vi "Linecut Example.vi"() -> ()   [LabVIEW 2016, in "graph_utilities.lvclass"]
uses:
  graph_utilities.lvclass
  graph_utilities.lvclass/graph_utilities.ctl
panel:
  in  "OK":bool
  in  "width (horizontal) 2":dbl=0.2
  in  "width (vertical) 2":dbl=0.2
  out "Horizontal 2":cluster{"Array":dbl[], "A x Vector":dbl[]}[](graph)
  out "Vertical 2":cluster{"Array":dbl[], "A x Vector":dbl[]}[](graph)
  in  "V2f 2":dbl[][](graph)=array73x213[15549 elements]
  in  "width (horizontal)":dbl=0.2
  in  "width (vertical)":dbl=0.2
  out "Horizontal":cluster{"Intensity Data":dbl[], "Array":dbl[]}[](graph)
  out "Vertical":cluster{"Array":dbl[], "A x Vector":dbl[]}[](graph)
  in  "V2f":dbl[][](graph)=array73x221[16133 elements]
  # "Control Graph:"
  # "Target:"
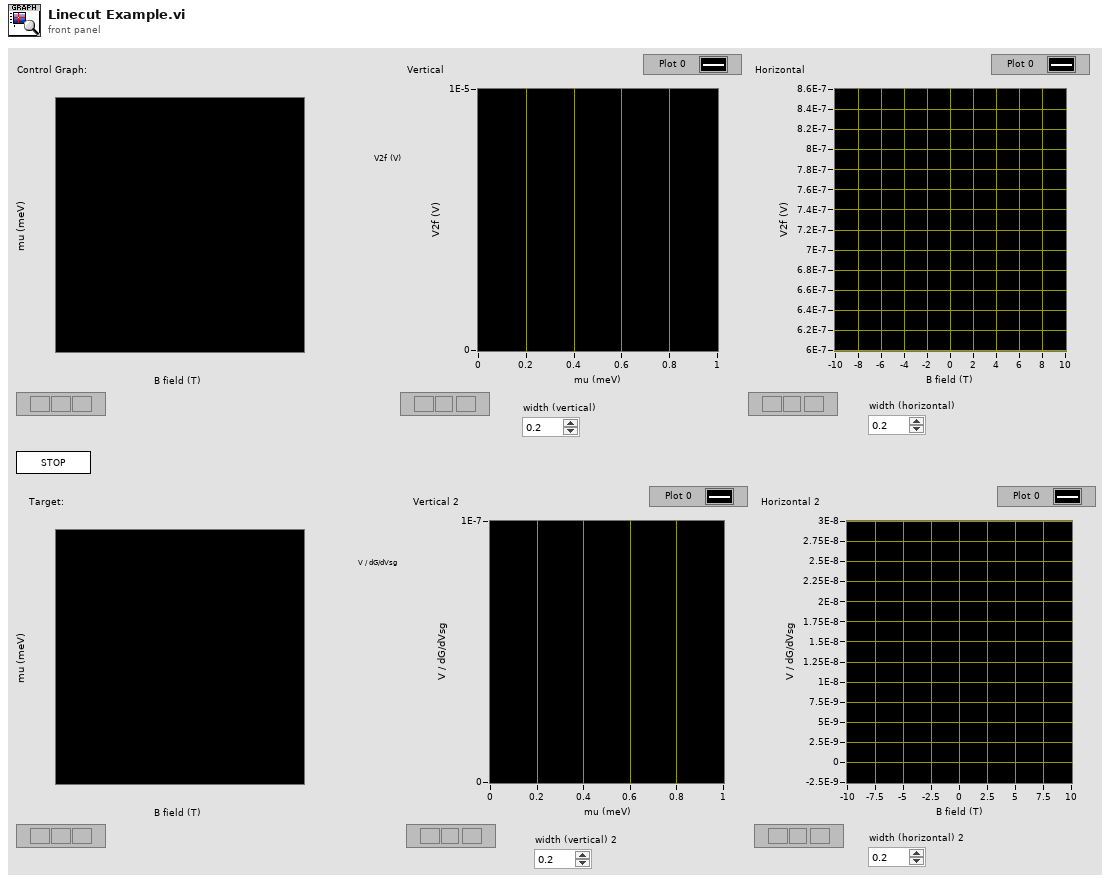
[diagram p1: front panel]
types:
  T1 = enum32{"Invalid", "Standard", "Closed", "Hidden", "Minimized", "Maximized"}
  T2 = enum32{"invalid app kind", "Development System", "Run Time System", "Student Edition", "Embedded LabVIEW", "Evaluation", "Custom"}
  T3 = cluster{"Core":cluster{"Current VI Reference":refnum<vi>, "Close Panel on Exit?":bool}, "graphs":refnum<class "graph_utilities.lvclass">[]}
  T4 = cluster{"Current VI Reference":refnum<vi>, "Close Panel on Exit?":bool}
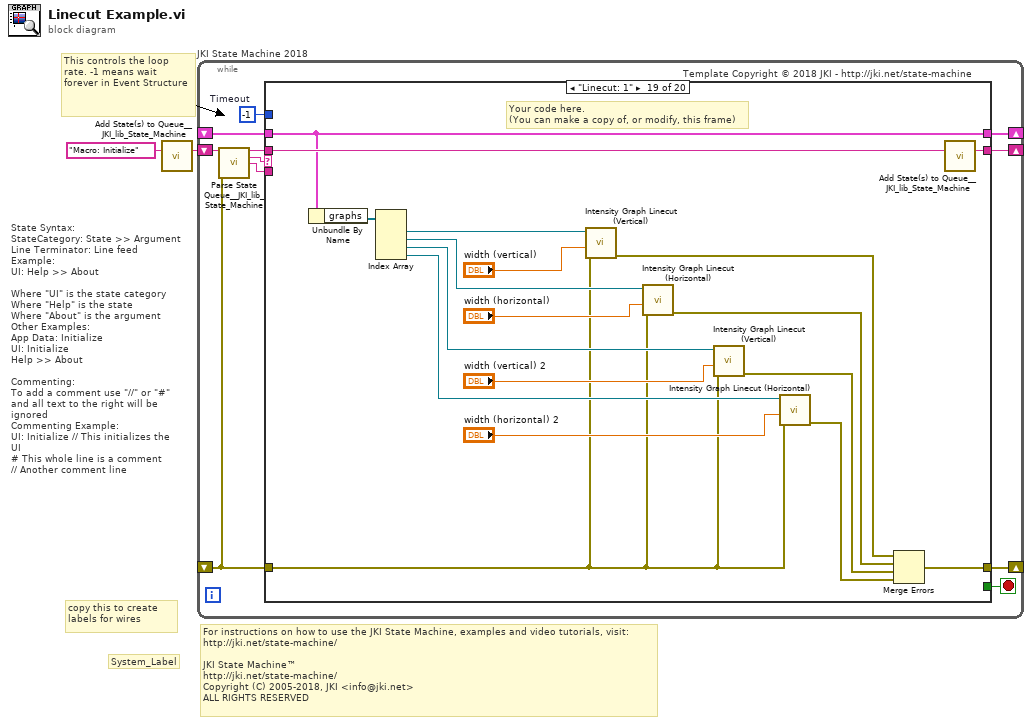
[diagram p0: block diagram]
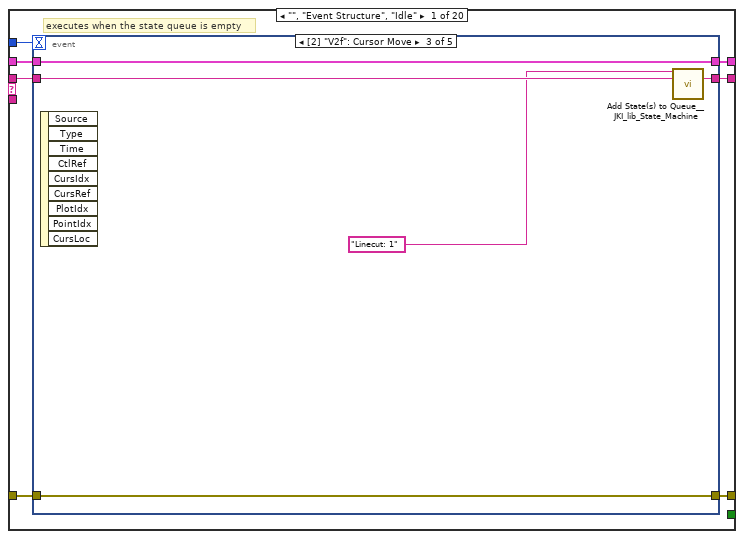
[diagram p2: hidden frame]
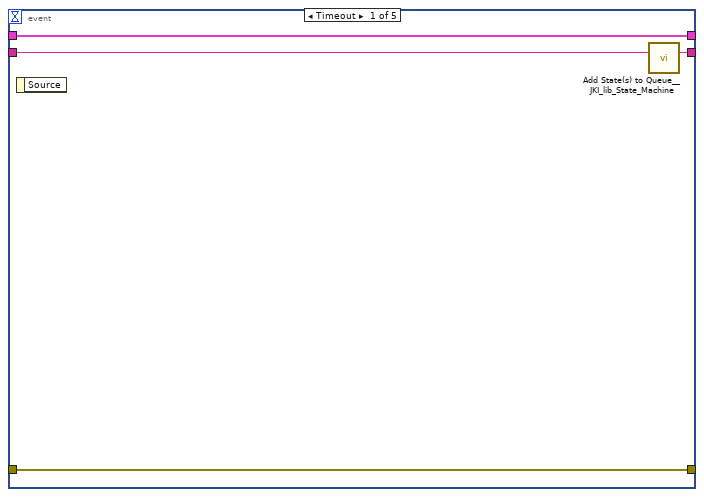
[diagram p3: hidden frame]
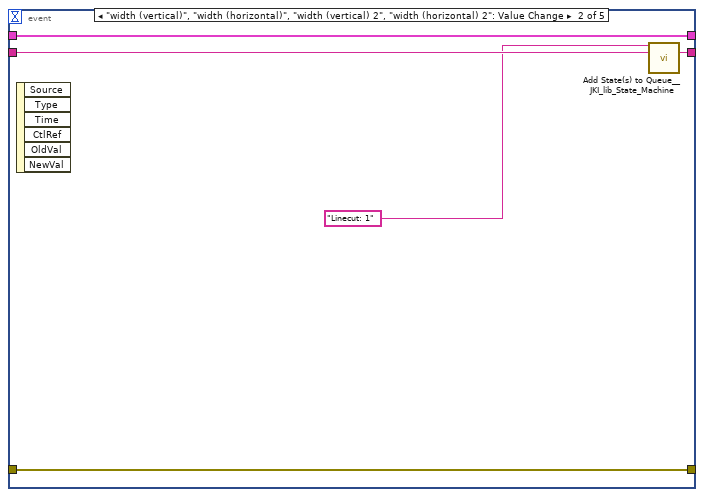
[diagram p4: hidden frame]
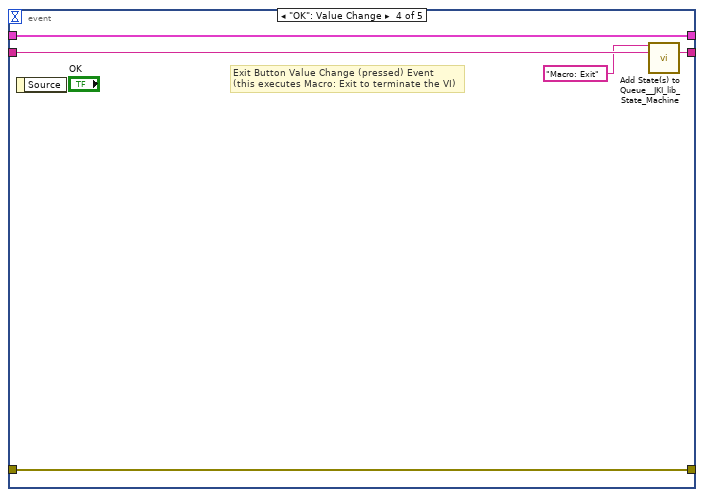
[diagram p5: hidden frame]
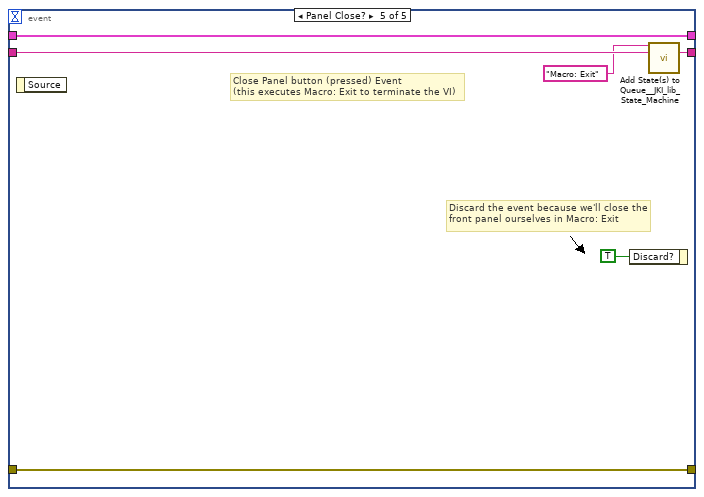
[diagram p6: hidden frame]
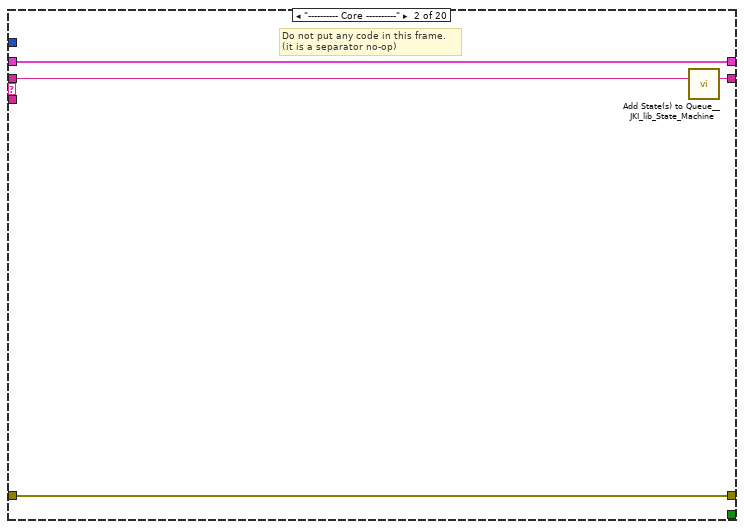
[diagram p7: hidden frame]
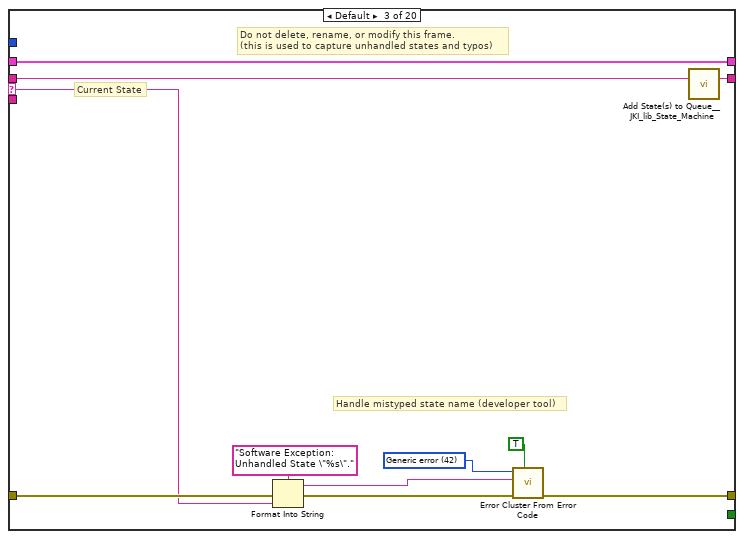
[diagram p8: hidden frame]
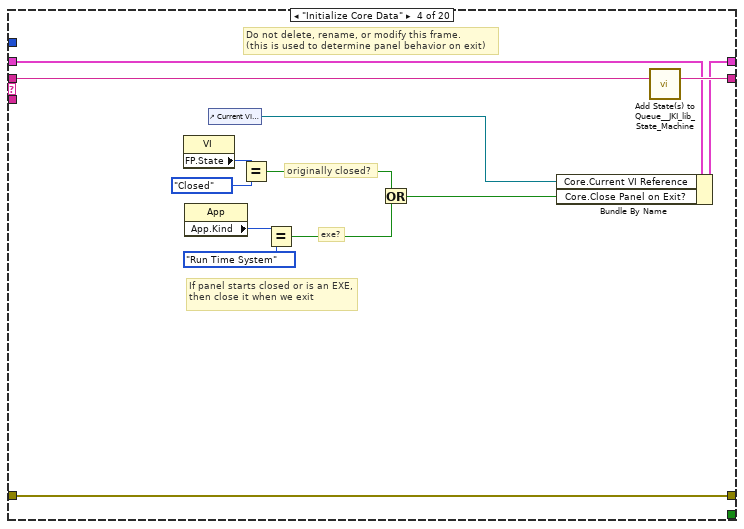
[diagram p9: hidden frame]
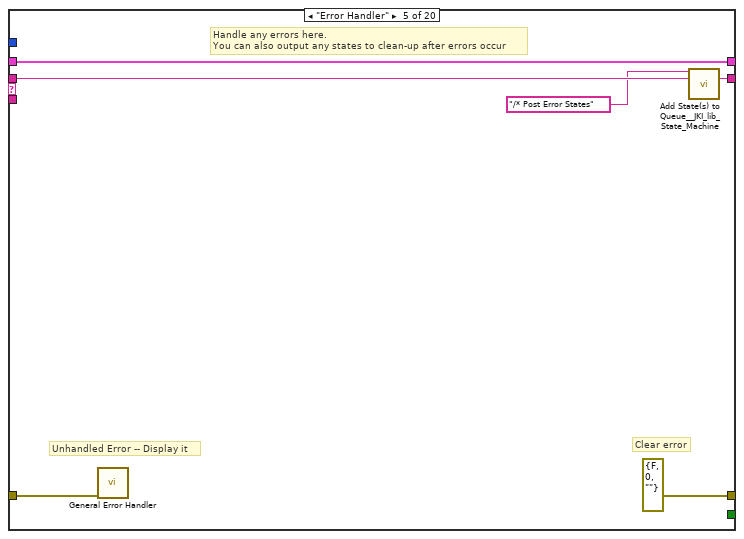
[diagram p10: hidden frame]
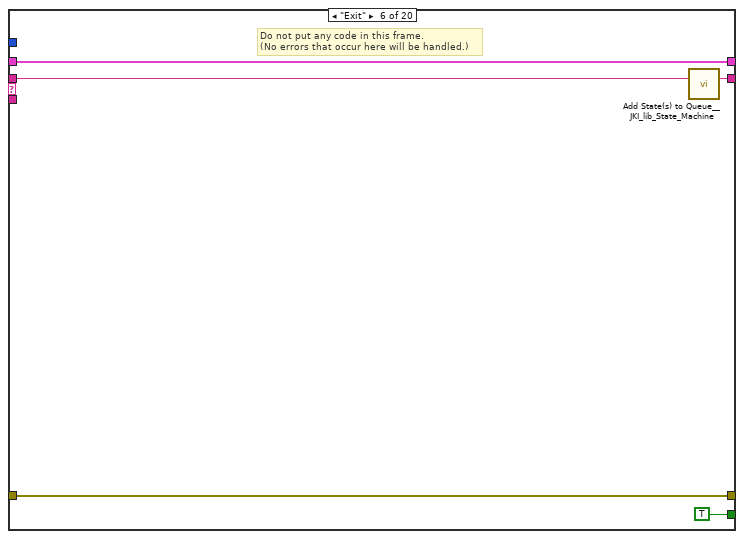
[diagram p11: hidden frame]
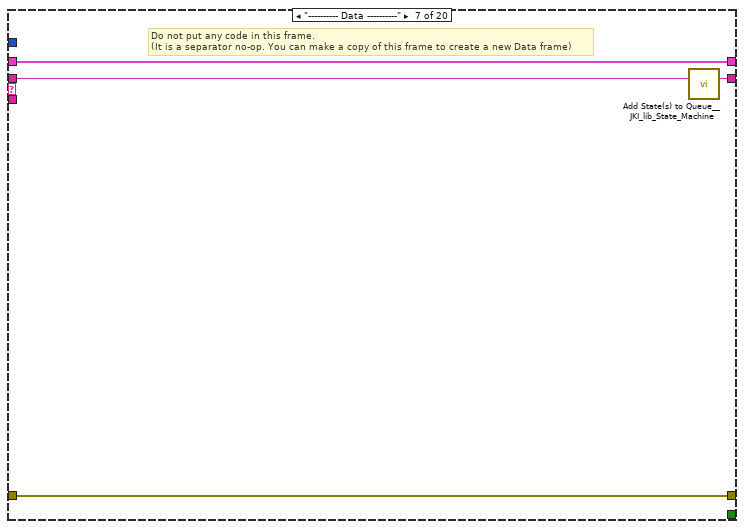
[diagram p12: hidden frame]
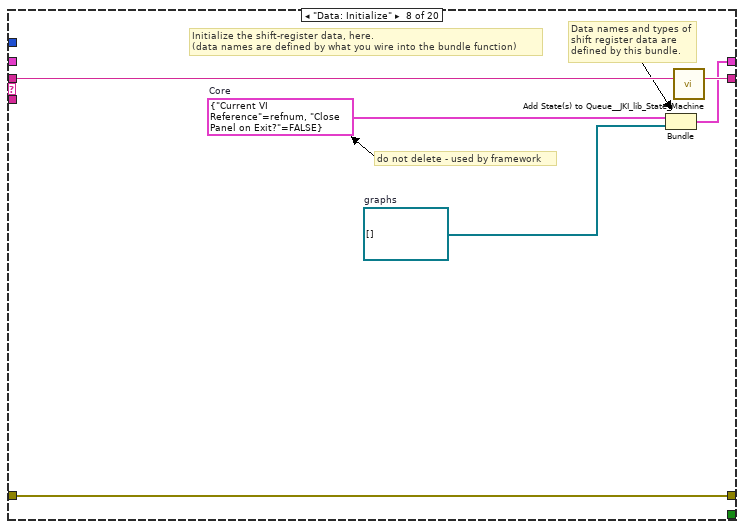
[diagram p13: hidden frame]
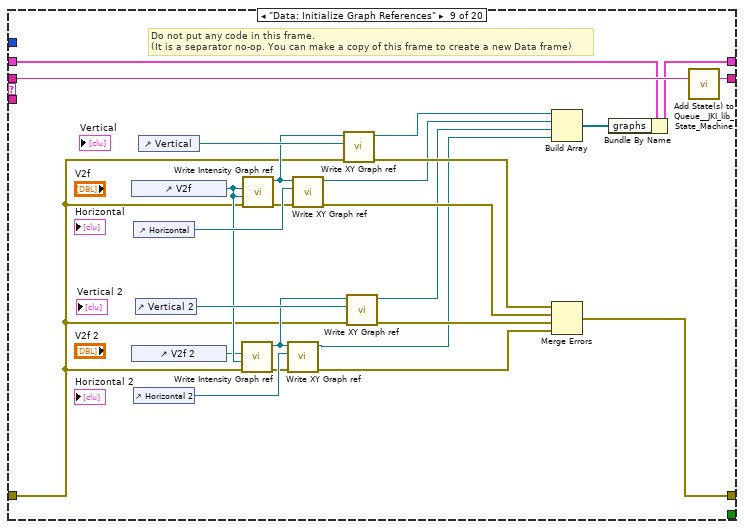
[diagram p14: hidden frame]
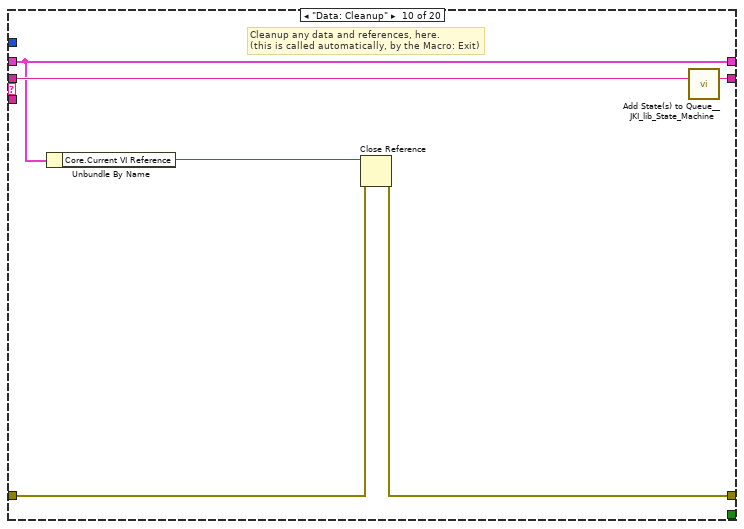
[diagram p15: hidden frame]
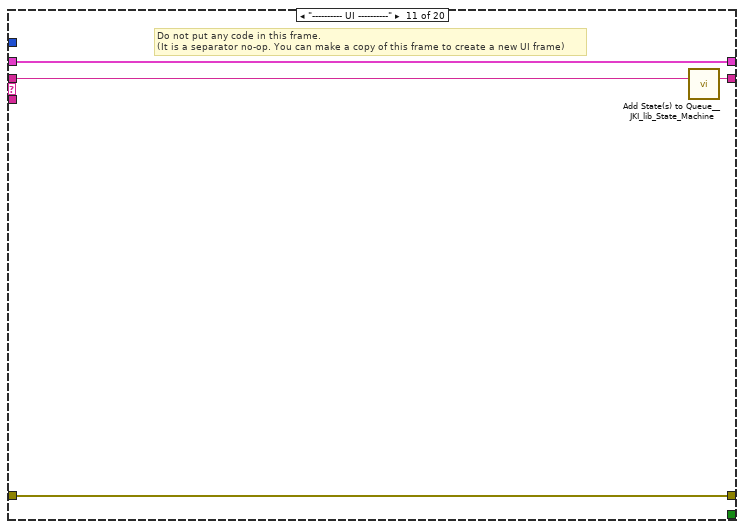
[diagram p16: hidden frame]
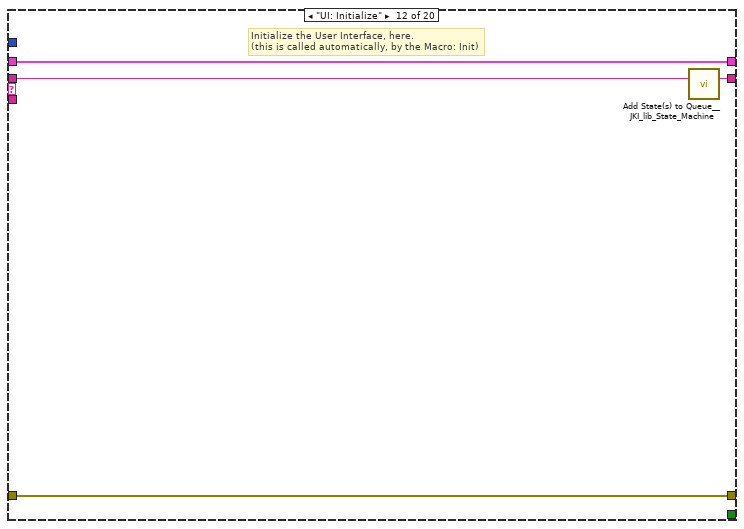
[diagram p17: hidden frame]
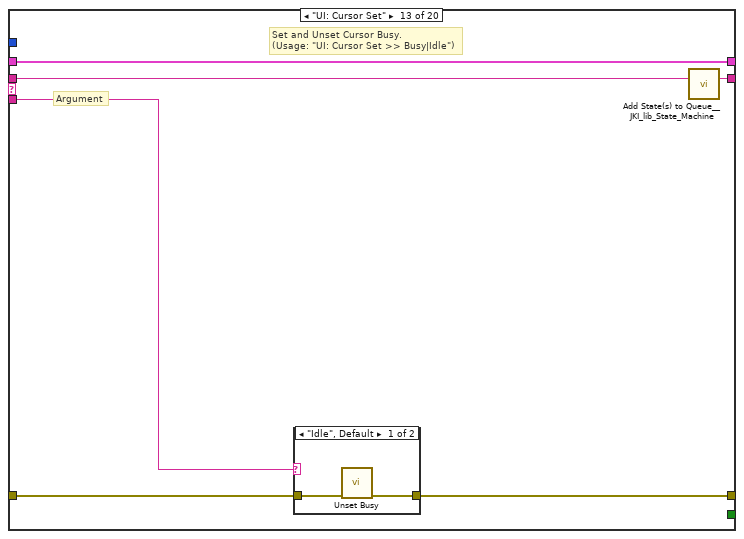
[diagram p18: hidden frame]
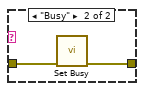
[diagram p19: hidden frame]
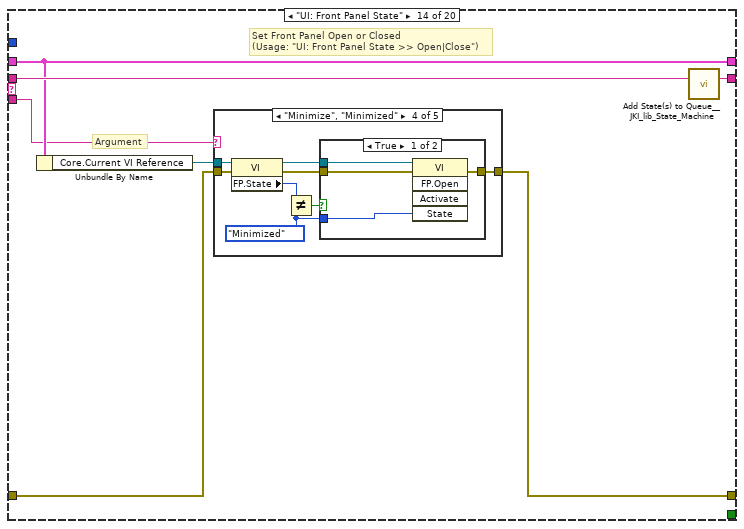
[diagram p20: hidden frame]
diagram:
  # "For instructions on how to use the JKI State Machine, examples and video tutorials, visit:\nhttp://jki.net/state-machine/\n\nJKI State Machine™\nhttp://jki.net/state-machine/\nCopyright (C) 2005-2018, JKI <info@jki.net>\nALL RIGHTS RESERVED"
  # "State Syntax:\nStateCategory: State >> Argument\nLine Terminator: Line feed\nExample:\nUI: Help >> About\n\nWhere \"UI\" is the state category\nWhere \"Help\" is the state\nWhere \"About\" is the argument\nOther Examples:\nApp Data: Initialize\nUI: Initialize\nHelp >> About\n\nCommenting:\nTo add a comment use \"//\" or \"#\" and all text to the right will be ignored\nCommenting Example:\nUI: Initialize // This initializes the UI\n# This whole line is a comment\n// Another comment line"
  # "copy this to create labels for wires"
  # "This controls the loop rate. -1 means wait forever in Event Structure"
  # "System_Label"
  n1 = call <vilib>:"Add State(s) to Queue__JKI_lib_State_Machine.vi"("State(s) in (\"\")"="Macro: Initialize") -> ("States Out"=w2:string)  [unwired: 14 in]
  n2 = while "JKI State Machine 2018" {
    shift-right: [w6] -> _
    shift-left: _ -> [w5]
    shift-right: [w9] -> _
    shift-left: _ -> [w3]
    shift-right: [w8] -> _
    shift-left: w2 -> [w10]
    stop <- w7 stop-if-true
    w4 = -1  # Timeout
    # "Template Copyright © 2018 JKI - http://jki.net/state-machine"
    n3 = call <vilib>:"Parse State Queue__JKI_lib_State_Machine.vi"("State Queue"=w10, "Error In (no error)"=w3) -> ("Remaining States"=w12:string, "Current State"=w13:string, "Arguments"=w11:string)  [unwired: 11 in]
    n4 = case shown="\"Linecut: 1\"" w13 {
      selector: w13 -> [_ _ w50 _ _ _ _ _ _ _ _ _ _ _ _ _ _ _ _ _]
      tunnel: w12 -> [w20 w49 w54 w73 w79 w84 w88 w94 w119 w125 w129 w133 w139 w150 w219 w225 w235 w239 w257 w261]
      tunnel: w11 -> [_ _ _ _ _ _ _ _ _ _ _ _ w134 w144 _ _ _ _ _ _]
      tunnel: w5 -> [w18 w46 w52 w66 w76 w82 w85 _ w103 w120 w126 w131 w137 w146 w216 w222 w232 w236 w251 w258]
      tunnel: [w17 w47 w56 w70 errorcluster {"status"=FALSE, "code"=0, "source"=""} ("error out") w81 w86 w91 w96 w121 w127 w130 w135 w147 w217 w223 w233 w237 w240 w259] -> w9
      tunnel: w3 -> [w16 w47 w55 w70 w75 w81 w86 w91 w95 w122 w127 w130 w136 w148 w217 w223 w233 w237 w241 w259]
      tunnel: [w19 w48 w53 w72 w78 w83 w87 w93 w118 w124 w128 w132 w138 w149 w218 w224 w234 w238 w256 w260] -> w8
      tunnel: [_ _ _ _ _ TRUE _ _ _ _ _ _ _ _ _ _ _ _ _ _] -> w7
      tunnel: [w15 w46 w52 w71 w76 w82 w85 w92 w102 w120 w126 w131 w137 w146 w216 w222 w232 w236 w251 w258] -> w6
      tunnel: w4 -> [w14 _ _ _ _ _ _ _ _ _ _ _ _ _ _ _ _ _ _ _]
      frame "", "Event Structure", "Idle" {
        # "executes when the state queue is empty"
        n5 = event shown="[2] \"V2f\": Cursor Move" {
          selector: _ -> [_ _ _ _ _]
          dyn-events: _ -> [_ _ _ _ _]
          timeout: w14 -> [_ _ _ _ _]
          tunnel: w20 -> [w24 w29 w34 w39 w45]
          tunnel: [w23 w28 w33 w38 w44] -> w19
          tunnel: w18 -> [w21 w26 w31 w36 w42]
          tunnel: [w22 w27 w32 w37 w43] -> w17
          tunnel: w16 -> [w22 w27 w32 w37 w43]
          tunnel: [w21 w26 w31 w36 w42] -> w15
          event Timeout {
            n6 = event-data() -> ()  [unwired: 1 in, 1 out]
            n7 = call <vilib>:"Add State(s) to Queue__JKI_lib_State_Machine.vi"("State(s) in (\"\")"=w24) -> ("States Out"=w23:string)  [unwired: 14 in]
          }
          event "width (vertical)", "width (horizontal)", "width (vertical) 2", "width (horizontal) 2": Value Change {
            n8 = event-data() -> ()  [unwired: 1 in, 6 out]
            n9 = call <vilib>:"Add State(s) to Queue__JKI_lib_State_Machine.vi"("State(s) in Front (\"\")"="Linecut: 1" ("State(s) in Front (\"\")"), "State(s) in (\"\")"=w29) -> ("States Out"=w28:string)  [unwired: 13 in]
          }
          event "V2f": Cursor Move {
            n10 = event-data() -> ()  [unwired: 1 in, 9 out]
            n11 = call <vilib>:"Add State(s) to Queue__JKI_lib_State_Machine.vi"("State(s) in Front (\"\")"="Linecut: 1" ("State(s) in Front (\"\")"), "State(s) in (\"\")"=w34) -> ("States Out"=w33:string)  [unwired: 13 in]
          }
          event "OK": Value Change {
            # "Exit Button Value Change (pressed) Event\n(this executes Macro: Exit to terminate the VI)"
            n12 = event-data() -> ()  [unwired: 1 in, 1 out]
            n13 = call <vilib>:"Add State(s) to Queue__JKI_lib_State_Machine.vi"("State(s) in Front (\"\")"="Macro: Exit", "State(s) in (\"\")"=w39) -> ("States Out"=w38:string)  [unwired: 13 in]
          }
          event Panel Close? {
            # "Discard the event because we'll close the front panel ourselves in Macro: Exit"
            # "Close Panel button (pressed) Event\n(this executes Macro: Exit to terminate the VI)"
            n14 = event-data() -> ()  [unwired: 1 in, 1 out]
            n15 = event-data("Discard?"=TRUE) -> ()  [unwired: 1 in, 1 out]
            n16 = call <vilib>:"Add State(s) to Queue__JKI_lib_State_Machine.vi"("State(s) in Front (\"\")"="Macro: Exit", "State(s) in (\"\")"=w45) -> ("States Out"=w44:string)  [unwired: 13 in]
          }
        }
      }
      frame "---------- Core ----------" {
        # "Do not put any code in this frame.\n(it is a separator no-op)"
        n17 = call <vilib>:"Add State(s) to Queue__JKI_lib_State_Machine.vi"("State(s) in (\"\")"=w49) -> ("States Out"=w48:string)  [unwired: 14 in]
      }
      frame Default {
        w59 = 42 items=["No error", "Argument error", "Memory is full", "Out of zone", "End of file", "File already open", "Generic file I/O error", "File not found", "File permission error", "Disk is full", "Duplicate path", "Too many files open", "System feature not enabled", "Resource file not found", "Cannot add resource", "Resource not found", "Image not found", "Image memory error", "Pen does not exist", "Config type invalid", "Config token not found", "Config parse error", "Config memory error", "Bad external code format", "Bad external code offset", "External code not present", "Null window", "Destroy window error", "Null menu", "Print aborted", "Bad print record", "Print driver error", "Windows error during printing", "Memory error during printing", "Print dialog error", "Generic print error", "Invalid device refnum", "Device not found", "Device parameter error", "Device unit error", "Cannot open device", "Device call aborted", "Generic error", "Cancelled by user", "Object ID too low", "Object ID too high", "Object not in heap", "Unknown heap", "Unknown object (invalid DefProc)", "Unknown object (DefProc not in table)", "Message out of range", "Invalid (null) method", "Unknown message", "Manager call not supported", "Bad address", "Network operation in progress", "Network operation timed out", "Connection is busy", "Network attribute not supported", "Network error", "Address in use", "System out of memory", "Connection aborted", "Connection refused", "Not connected", "Already connected", "Connection closed", "Initialization error (interapplication manager)", "Bad occurrence", "Wait on unbound occurrence handler", "Occurrence queue overflow", "Datalog type conflict", "Unused", "Unrecognized type (interapplication manager)", "Memory corrupt", "Failed to make temporary DLL", "Old CIN version", "Drag socket not found", "Failed to load drop-object", "Failed to register OLE object", "Failed to release OLE object", "Format specifier type mismatch", "Unknown format specifier", "Too few format specifiers", "Too many format specifiers", "Scan failed", "Newer CIN version", "Error converting to variant", "Runtime menu error", "Password tampered", "Variant attribute not found", "Incompatible variant data type", "Event data is not available", "Event Store is not present", "Occurrence is not found", "Event Queue is not created", "Event info is not available", "Refnum passed is NULL", "Error retrieving Class GUID", "Error retrieving CoClass GUID", "Error retrieving TypeLib GUID.", "Bad built application magic bytes.", "Specific driver is different from the specific driver associated with the Logical Name.", "There is no session opened to the class driver.", "Max Error", "MAX - Error with config objects", "MAX - Error loading configuration", "MAX - Group not supported"]
        # "Current State"
        # "Do not delete, rename, or modify this frame.\n(this is used to capture unhandled states and typos)"
        # "Handle mistyped state name (developer tool)"
        n18 = Format Into String(format string="Software Exception: Unhandled State \"%s\"." ("message"), error in=w55, w50) -> (resulting string=w58:string, error out=w57:errorcluster)  [unwired: 1 in]
        n19 = call <vilib>:"Error Cluster From Error Code.vi"("show call chain? (False)"=TRUE, "error in (no error)"=w57, "error message (\"\")"=w58, "error code (0)"=w59) -> ("error out"=w56:errorcluster)  [unwired: 5 in]
        n20 = call <vilib>:"Add State(s) to Queue__JKI_lib_State_Machine.vi"("State(s) in (\"\")"=w54) -> ("States Out"=w53:string)  [unwired: 14 in]
      }
      frame "Initialize Core Data" {
        # "Do not delete, rename, or modify this frame.\n(this is used to determine panel behavior on exit)"
        # "originally closed?"
        # "exe?"
        # "If panel starts closed or is an EXE, then close it when we exit"
        n21 = property class="VI"() -> ("FP.State"=w63:T1)  [unwired: 2 in, 2 out]
        n22 = property class="App"() -> ("App.Kind"=w69:T2)  [unwired: 2 in, 2 out]
        n23 = control-ref of="Current VI Reference"() -> (w64:refnum<vi>)
        n24 = Equal?(x=w63, y=T1."Closed" ("Front Panel Window:State")) -> (x = y?=w61:bool)
        n25 = Equal?(x=w69, y=T2."Run Time System" ("Application:Kind")) -> (x = y?=w67:bool)
        n26 = Or(x=w61, y=w67) -> (x .or. y?=w65:bool)
        n27 = Bundle By Name(cluster=w66, "Core.Current VI Reference"=w64, "Core.Close Panel on Exit?"=w65) -> (w71:T3)
        n28 = call <vilib>:"Add State(s) to Queue__JKI_lib_State_Machine.vi"("State(s) in (\"\")"=w73) -> ("States Out"=w72:string)  [unwired: 14 in]
      }
      frame "Error Handler" {
        # "Unhandled Error -- Display it"
        # "Handle any errors here.\nYou can also output any states to clean-up after errors occur"
        # "Clear error"
        n29 = call <vilib>:"General Error Handler.vi"("error in (no error)"=w75) -> ()  [unwired: 10 in, 5 out]
        n30 = call <vilib>:"Add State(s) to Queue__JKI_lib_State_Machine.vi"("State(s) in Front (\"\")"="/* Post Error States", "State(s) in (\"\")"=w79) -> ("States Out"=w78:string)  [unwired: 13 in]
      }
      frame "Exit" {
        # "Do not put any code in this frame.\n(No errors that occur here will be handled.)"
        n31 = call <vilib>:"Add State(s) to Queue__JKI_lib_State_Machine.vi"("State(s) in (\"\")"=w84) -> ("States Out"=w83:string)  [unwired: 14 in]
      }
      frame "---------- Data ----------" {
        # "Do not put any code in this frame.\n(It is a separator no-op. You can make a copy of this frame to create a new Data frame)"
        n32 = call <vilib>:"Add State(s) to Queue__JKI_lib_State_Machine.vi"("State(s) in (\"\")"=w88) -> ("States Out"=w87:string)  [unwired: 14 in]
      }
      frame "Data: Initialize" {
        w89 = refnum<class "graph_utilities.lvclass">[] []  # graphs
        w90 = T4 {"Current VI Reference"=refnum, "Close Panel on Exit?"=FALSE}  # Core
        # "do not delete - used by framework"
        # "Data names and types of shift register data are defined by this bundle."
        # "Initialize the shift-register data, here.\n(data names are defined by what you wire into the bundle function)"
        n33 = Bundle("Core"=w90, "graphs"=w89) -> (w92:T3)  [unwired: 1 in]
        n34 = call <vilib>:"Add State(s) to Queue__JKI_lib_State_Machine.vi"("State(s) in (\"\")"=w94) -> ("States Out"=w93:string)  [unwired: 14 in]
      }
      frame "Data: Initialize Graph References" {
        # "Do not put any code in this frame.\n(It is a separator no-op. You can make a copy of this frame to create a new Data frame)"
        n35 = control-ref of="V2f"() -> (w109:refnum<vi>)
        n36 = control-ref of="V2f 2"() -> (w108:refnum<vi>)
        n37 = control-ref of="Horizontal"() -> (w111:refnum<vi>)
        n38 = control-ref of="Horizontal 2"() -> (w114:refnum<vi>)
        n39 = control-ref of="Vertical 2"() -> (w116:refnum<vi>)
        n40 = control-ref of="Vertical"() -> (w117:refnum<vi>)
        n41 = call "Write Intensity Graph ref.vi"("error in (no error)"=w95, "Intensity Graph (Control)"=w109, "Intensity Graph"=w108) -> ("error out"=w113:errorcluster, "graph_utilities out"=w115:refnum<class "graph_utilities.lvclass">)  [unwired: 7 in]
        n42 = call "Write Intensity Graph ref.vi"("error in (no error)"=w95, "Intensity Graph (Control)"=w109, "Intensity Graph"=w109) -> ("error out"=w110:errorcluster, "graph_utilities out"=w112:refnum<class "graph_utilities.lvclass">)  [unwired: 7 in]
        n43 = call "Write XY Graph ref.vi"("error in (no error)"=w113, "XY Graph"=w114, "graph_utilities in"=w115) -> ("error out"=w107:errorcluster, "graph_utilities out"=w98:refnum<class "graph_utilities.lvclass">)  [unwired: 7 in]
        n44 = call "Write XY Graph ref.vi"("error in (no error)"=w110, "XY Graph"=w111, "graph_utilities in"=w112) -> ("error out"=w105:errorcluster, "graph_utilities out"=w100:refnum<class "graph_utilities.lvclass">)  [unwired: 7 in]
        n45 = call "Write XY Graph ref.vi"("error in (no error)"=w95, "XY Graph"=w117, "graph_utilities in"=w112) -> ("error out"=w104:errorcluster, "graph_utilities out"=w101:refnum<class "graph_utilities.lvclass">)  [unwired: 7 in]
        n46 = call "Write XY Graph ref.vi"("error in (no error)"=w95, "XY Graph"=w116, "graph_utilities in"=w115) -> ("error out"=w106:errorcluster, "graph_utilities out"=w99:refnum<class "graph_utilities.lvclass">)  [unwired: 7 in]
        n47 = Build Array(w101, w100, w99, w98) -> (w97:refnum<class "graph_utilities.lvclass">[])
        n48 = Merge Errors(w104, w105, w106, w107) -> (w96:errorcluster)
        n49 = Bundle By Name(cluster=w103, "graphs"=w97) -> (w102:T3)
        n50 = call <vilib>:"Add State(s) to Queue__JKI_lib_State_Machine.vi"("State(s) in (\"\")"=w119) -> ("States Out"=w118:string)  [unwired: 14 in]
      }
      frame "Data: Cleanup" {
        # "Cleanup any data and references, here.\n(this is called automatically, by the Macro: Exit)"
        n51 = Unbundle By Name(w120) -> ("Core.Current VI Reference"=w123:refnum<vi>)
        n52 = Close Reference(reference=w123, error in (no error)=w122) -> (error out=w121:errorcluster)
        n53 = call <vilib>:"Add State(s) to Queue__JKI_lib_State_Machine.vi"("State(s) in (\"\")"=w125) -> ("States Out"=w124:string)  [unwired: 14 in]
      }
      frame "---------- UI ----------" {
        # "Do not put any code in this frame.\n(It is a separator no-op. You can make a copy of this frame to create a new UI frame)"
        n54 = call <vilib>:"Add State(s) to Queue__JKI_lib_State_Machine.vi"("State(s) in (\"\")"=w129) -> ("States Out"=w128:string)  [unwired: 14 in]
      }
      frame "UI: Initialize" {
        # "Initialize the User Interface, here.\n(this is called automatically, by the Macro: Init)"
        n55 = call <vilib>:"Add State(s) to Queue__JKI_lib_State_Machine.vi"("State(s) in (\"\")"=w133) -> ("States Out"=w132:string)  [unwired: 14 in]
      }
      frame "UI: Cursor Set" {
        # "Argument"
        # "Set and Unset Cursor Busy.\n(Usage: \"UI: Cursor Set >> Busy|Idle\")"
        n56 = case shown="\"Idle\", Default" w134 {
          tunnel: w136 -> [w141 w143]
          tunnel: [w140 w142] -> w135
          frame "Idle", Default {
            n57 = call <vilib>:"Unset Busy.vi"("error in (no error)"=w141) -> ("error out"=w140:errorcluster)  [unwired: 10 in]
          }
          frame "Busy" {
            n58 = call <vilib>:"Set Busy.vi"("error in (no error)"=w143) -> ("error out"=w142:errorcluster)  [unwired: 9 in, 1 out]
          }
        }
        n59 = call <vilib>:"Add State(s) to Queue__JKI_lib_State_Machine.vi"("State(s) in (\"\")"=w139) -> ("States Out"=w138:string)  [unwired: 14 in]
      }
      frame "UI: Front Panel State" {
        # "Argument"
        # "Set Front Panel Open or Closed\n(Usage: \"UI: Front Panel State >> Open|Close\")"
        n60 = Unbundle By Name(w146) -> ("Core.Current VI Reference"=w145:refnum<vi>)
        n61 = case shown="\"Minimize\", \"Minimized\"" w144 {
          tunnel: w148 -> [w156 w171 w182 w195 w208]
          tunnel: [w158 w172 w184 w197 w210] -> w147
          tunnel: w145 -> [w157 w169 w183 w196 w209]
          frame "Open", "Standard", Default {
            w151 = T1."Standard" ("State")
            n62 = property class="VI"(reference=w157, error in=w156) -> (reference out=w154:refnum<vi>, error out=w155:errorcluster, "FP.State"=w153:T1)
            n63 = Not Equal?(x=w153, y=w151) -> (x != y?=w152:bool)
            n64 = case shown="True" w152 {
              tunnel: [w162 w164] -> w158
              tunnel: w155 -> [w161 w164]
              tunnel: w154 -> [w160 _]
              tunnel: w151 -> [w159 _]
              frame True {
                n65 = invoke class="VI" method="FP.Open"(reference=w160, error in=w161, "Activate"=TRUE, "State"=w159) -> (error out=w162:errorcluster)  [unwired: 1 in, 4 out]
              }
              frame False {
              }
            }
          }
          frame "Close", "Closed" {
            n66 = property class="VI"(reference=w169, error in=w171) -> (reference out=w168:refnum<vi>, error out=w170:errorcluster, "FP.State"=w166:T1)
            n67 = Not Equal?(x=w166, y=T1."Closed" ("Front Panel Window:State")) -> (x != y?=w165:bool)
            n68 = case shown="True" w165 {
              tunnel: [w173 w176] -> w172
              tunnel: w170 -> [w173 w175]
              tunnel: w168 -> [_ w174]
              frame False {
              }
              frame True {
                n69 = invoke class="VI" method="FP.Close"(reference=w174, error in=w175) -> (error out=w176:errorcluster)  [unwired: 1 in, 2 out]
              }
            }
          }
          frame "Hidden", "Hide" {
            w177 = T1."Hidden" ("State")
            n70 = property class="VI"(reference=w183, error in=w182) -> (reference out=w180:refnum<vi>, error out=w181:errorcluster, "FP.State"=w179:T1)
            n71 = Not Equal?(x=w179, y=w177) -> (x != y?=w178:bool)
            n72 = case shown="True" w178 {
              tunnel: [w188 w189] -> w184
              tunnel: w181 -> [w187 w189]
              tunnel: w180 -> [w186 _]
              tunnel: w177 -> [w185 _]
              frame True {
                n73 = invoke class="VI" method="FP.Open"(reference=w186, error in=w187, "State"=w185) -> (error out=w188:errorcluster)  [unwired: 2 in, 4 out]
              }
              frame False {
              }
            }
          }
          frame "Minimize", "Minimized" {
            w190 = T1."Minimized" ("State")
            n74 = property class="VI"(reference=w196, error in=w195) -> (reference out=w193:refnum<vi>, error out=w194:errorcluster, "FP.State"=w192:T1)
            n75 = Not Equal?(x=w192, y=w190) -> (x != y?=w191:bool)
            n76 = case shown="True" w191 {
              tunnel: [w201 w202] -> w197
              tunnel: w194 -> [w200 w202]
              tunnel: w193 -> [w199 _]
              tunnel: w190 -> [w198 _]
              frame True {
                n77 = invoke class="VI" method="FP.Open"(reference=w199, error in=w200, "State"=w198) -> (error out=w201:errorcluster)  [unwired: 2 in, 4 out]
              }
              frame False {
              }
            }
          }
          frame "Maximize", "Maximized" {
            w203 = T1."Maximized" ("State")
            n78 = property class="VI"(reference=w209, error in=w208) -> (reference out=w206:refnum<vi>, error out=w207:errorcluster, "FP.State"=w205:T1)
            n79 = Not Equal?(x=w205, y=w203) -> (x != y?=w204:bool)
            n80 = case shown="True" w204 {
              tunnel: [w214 w215] -> w210
              tunnel: w207 -> [w213 w215]
              tunnel: w206 -> [w212 _]
              tunnel: w203 -> [w211 _]
              frame True {
                n81 = invoke class="VI" method="FP.Open"(reference=w212, error in=w213, "State"=w211) -> (error out=w214:errorcluster)  [unwired: 2 in, 4 out]
              }
              frame False {
              }
            }
          }
        }
        n82 = call <vilib>:"Add State(s) to Queue__JKI_lib_State_Machine.vi"("State(s) in (\"\")"=w150) -> ("States Out"=w149:string)  [unwired: 14 in]
      }
      frame "---------- Macro ----------" {
        # "Do not put any code in this frame.\n(It is a separator no-op. You can make a copy of this frame to create a new Macro frame)"
        n83 = call <vilib>:"Add State(s) to Queue__JKI_lib_State_Machine.vi"("State(s) in (\"\")"=w219) -> ("States Out"=w218:string)  [unwired: 14 in]
      }
      frame "Macro: Initialize" {
        w221 = "Data: Initialize\nInitialize Core Data\nUI: Initialize\nUI: Front Panel State >> Open"  # Data: Initialize Initialize Core Data UI: Initialize UI: Front Panel State >> Open
        # "Initialization Macro\n(This is called once, when the VI starts)"
        n84 = call <vilib>:"Add State(s) to Queue__JKI_lib_State_Machine.vi"("State(s) in Front (\"\")"=w221, "State(s) in (\"\")"=w225, "State(s) at Back (\"\")"="Data: Initialize Graph References\nLinecut: 1") -> ("States Out"=w224:string)  [unwired: 12 in]
      }
      frame "Macro: Exit" {
        # "Exit Macro\n(This is called once, when the VI exits)"
        n85 = Unbundle By Name(w232) -> ("Core.Close Panel on Exit?"=w231:bool)
        n86 = Select(t="UI: Front Panel State >> Close", s=w231, f="") -> (s? t:f=w228:string)
        n87 = call <vilib>:"Add State(s) to Queue__JKI_lib_State_Machine.vi"("State(s) in (\"\")"=w228, "State(s) at Back (\"\")"="Data: Cleanup\nExit") -> ("States Out"=w226:string)  [unwired: 13 in]
        n88 = call <vilib>:"Add State(s) to Queue__JKI_lib_State_Machine.vi"("State(s) in Front (\"\")"=w226, "State(s) in (\"\")"=w235) -> ("States Out"=w234:string)  [unwired: 13 in]
      }
      frame "---------- Linecut ----------" {
        # "Template Separator\n(You can make a copy of, or modify, this frame)"
        n89 = call <vilib>:"Add State(s) to Queue__JKI_lib_State_Machine.vi"("State(s) in (\"\")"=w239) -> ("States Out"=w238:string)  [unwired: 14 in]
      }
      frame "Linecut: 1" {
        # "Your code here.\n(You can make a copy of, or modify, this frame)"
        n90 = Unbundle By Name(w251) -> ("graphs"=w250:refnum<class "graph_utilities.lvclass">[])
        n91 = Index Array(array=w250) -> (element #1=w249:refnum<class "graph_utilities.lvclass">, element #2=w248:refnum<class "graph_utilities.lvclass">, element #3=w247:refnum<class "graph_utilities.lvclass">, element #4=w246:refnum<class "graph_utilities.lvclass">)  [unwired: 4 in]
        n92 = call "Intensity Graph Linecut (Vertical).vi"("error in (no error)"=w241, "width (vertical)"="width (vertical)", "graph_utilities in"=w249) -> ("error out"=w245:errorcluster)  [unwired: 7 in, 1 out]
        n93 = call "Intensity Graph Linecut (Horizontal).vi"("error in (no error)"=w241, "width (horizontal)"="width (horizontal)", "graph_utilities in"=w248) -> ("error out"=w244:errorcluster)  [unwired: 7 in, 1 out]
        n94 = call "Intensity Graph Linecut (Vertical).vi"("error in (no error)"=w241, "width (vertical)"="width (vertical) 2", "graph_utilities in"=w247) -> ("error out"=w243:errorcluster)  [unwired: 7 in, 1 out]
        n95 = call "Intensity Graph Linecut (Horizontal).vi"("error in (no error)"=w241, "width (horizontal)"="width (horizontal) 2", "graph_utilities in"=w246) -> ("error out"=w242:errorcluster)  [unwired: 7 in, 1 out]
        n96 = Merge Errors(w245, w244, w243, w242) -> (w240:errorcluster)
        n97 = call <vilib>:"Add State(s) to Queue__JKI_lib_State_Machine.vi"("State(s) in (\"\")"=w257) -> ("States Out"=w256:string)  [unwired: 14 in]
      }
      frame "Linecut: 2" {
        # "Your code here.\n(You can make a copy of, or modify, this frame)"
        n98 = call <vilib>:"Add State(s) to Queue__JKI_lib_State_Machine.vi"("State(s) in (\"\")"=w261) -> ("States Out"=w260:string)  [unwired: 14 in]
      }
    }
  }
